vi "外观 2.vi"(0 "Data In":T4 caption="数据输入", 2 "Display State In":T2 caption="显示状态输入", 3 "Container State":T3 caption="容器状态") -> (6 "Data Out":T4 caption="数据输出", 7 "Display State Out":T2 caption="显示状态输出", 8 "Action":T1 caption="动作")   [LabVIEW 2016, in "多参数测量数据.xctl"]
uses:
  <vilib>/_xctls/Container State.ctl
  <vilib>/_xctls/Action.ctl
  <vilib>/_xctls/XControlSupport.lvlib
panel:
  out "数据标识":string
  out "实测值":string
  out "数据时间":string
  out "单位":string
  out "因子编码":string
  # "因子编码:"
  # "单位:"
  # "数据时间:"
  # "实测值:"
  # "数据标识:"
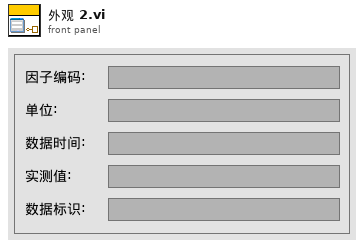
[diagram p1: front panel]
types:
  T1 = typedef "XControlSupport.lvlib/Action.ctl" = cluster{"Data Changed?":bool, "State Changed?":bool, "Action Name":string}
  T2 = typedef "多参数测量数据.xctl/状态 1.ctl" = cluster{"Numeric":dbl}
  T3 = typedef "XControlSupport.lvlib/Container State.ctl" = cluster{"Indicator?":bool, "Run Mode?":bool, " Refnum":refnum<vi>}
  T4 = typedef "多参数测量数据.xctl/数据 1.ctl" = cluster{"测量精度":u16, "测量数据区":cluster{"因子编码":string, "单位":string, "标样参考值":sgl, "水样数据时间":timestamp, "水样实测值":sgl, "水样数据标识":string, "K":sgl, "B":sgl, "T":sgl, "H":sgl, "水深":sgl}}
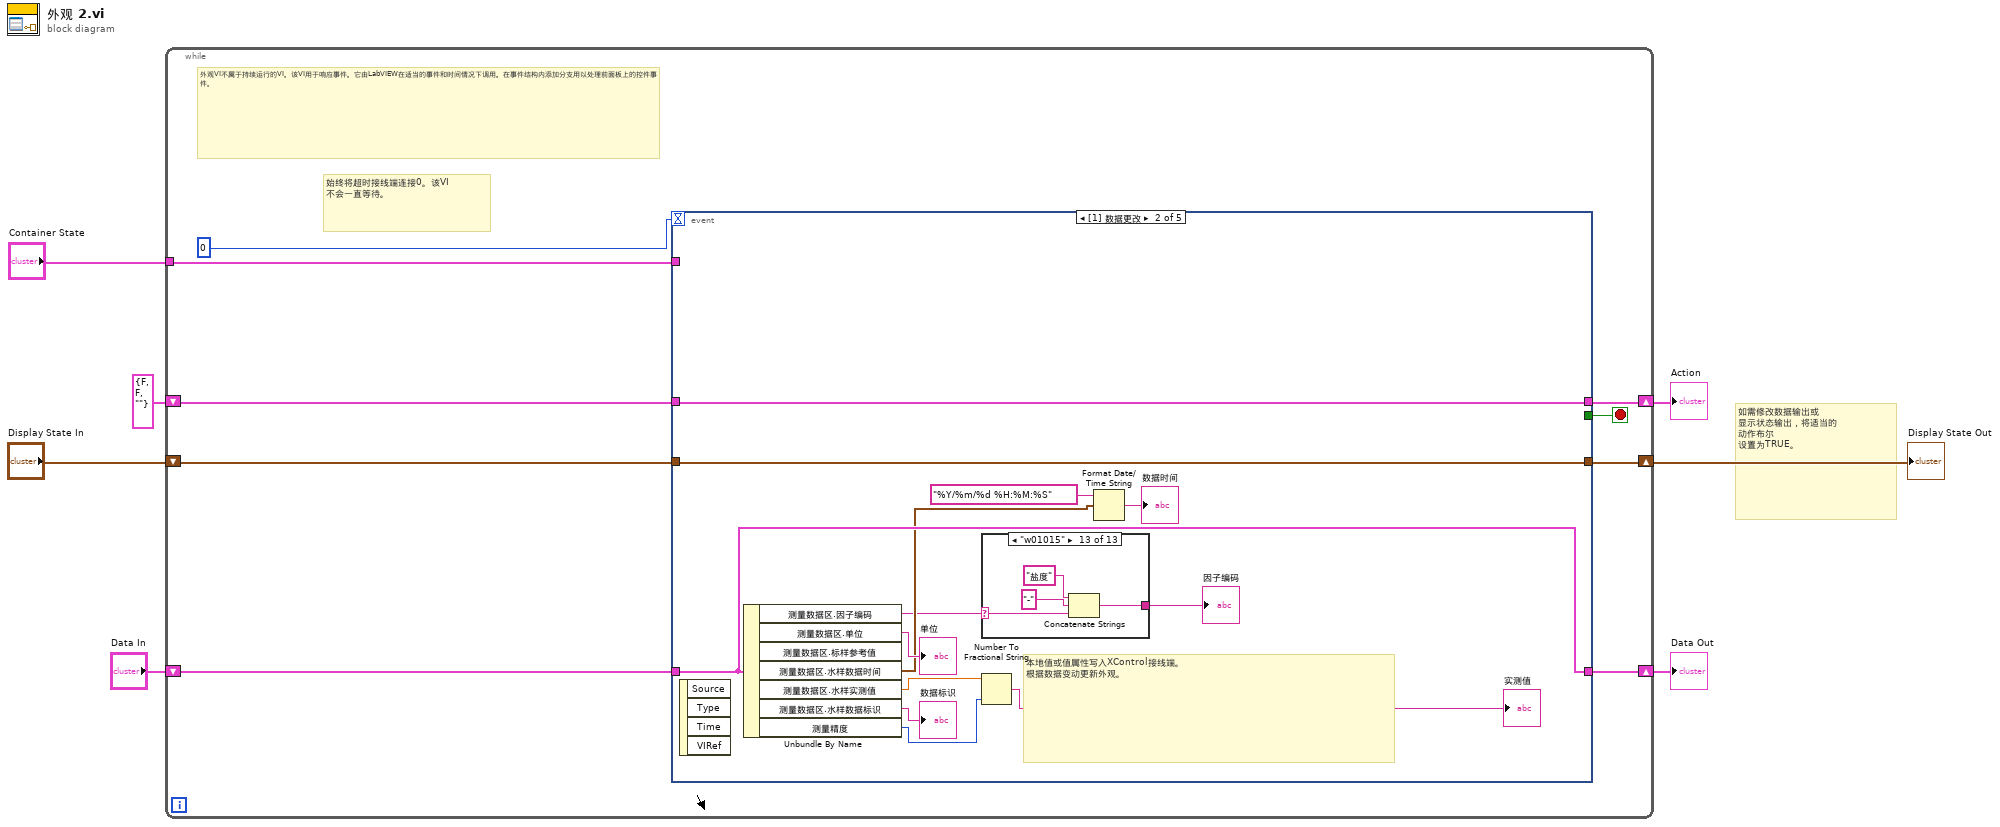
[diagram p0: block diagram]
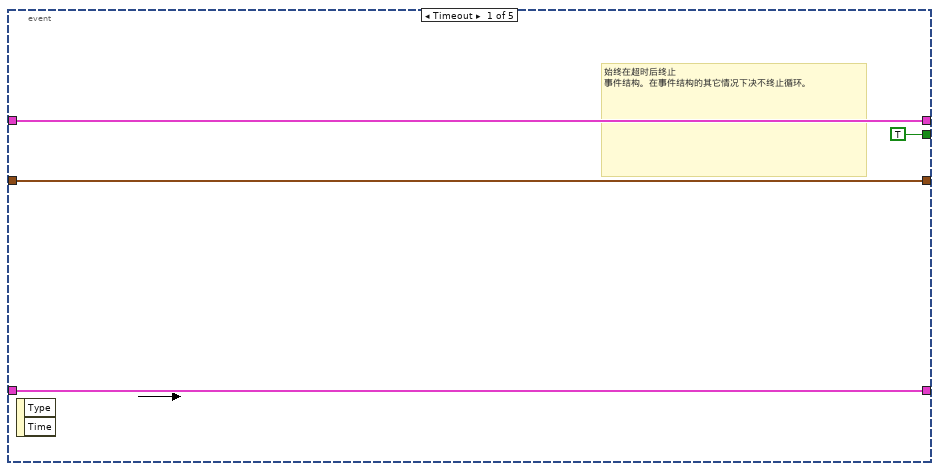
[diagram p2: hidden frame]
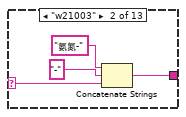
[diagram p4: hidden frame]
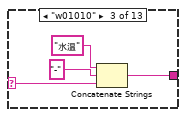
[diagram p5: hidden frame]
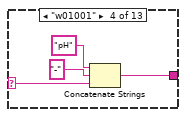
[diagram p6: hidden frame]
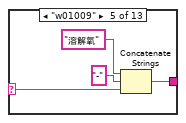
[diagram p7: hidden frame]
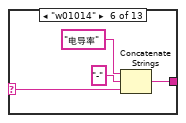
[diagram p8: hidden frame]
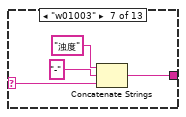
[diagram p9: hidden frame]
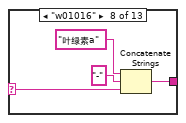
[diagram p10: hidden frame]
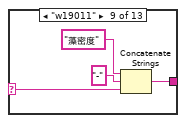
[diagram p11: hidden frame]
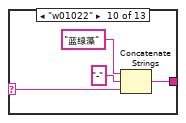
[diagram p12: hidden frame]
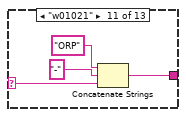
[diagram p13: hidden frame]
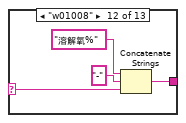
[diagram p14: hidden frame]
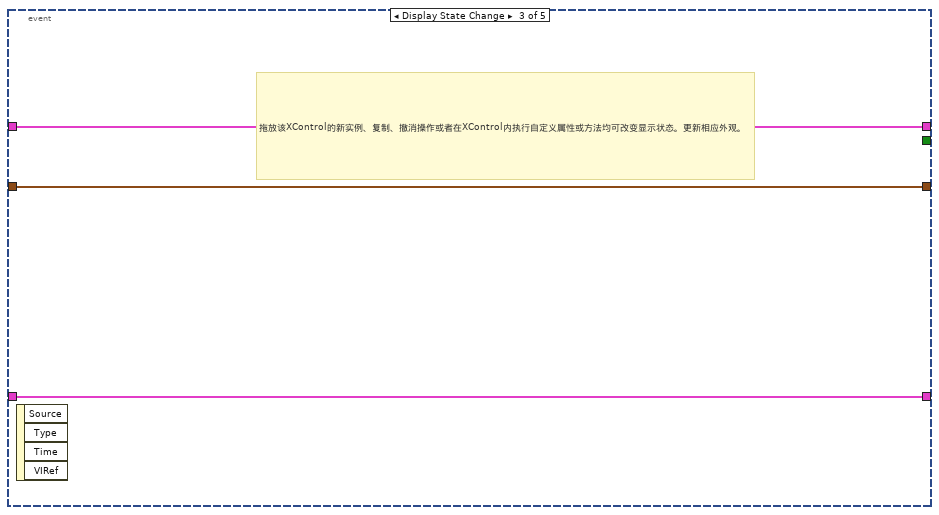
[diagram p15: hidden frame]
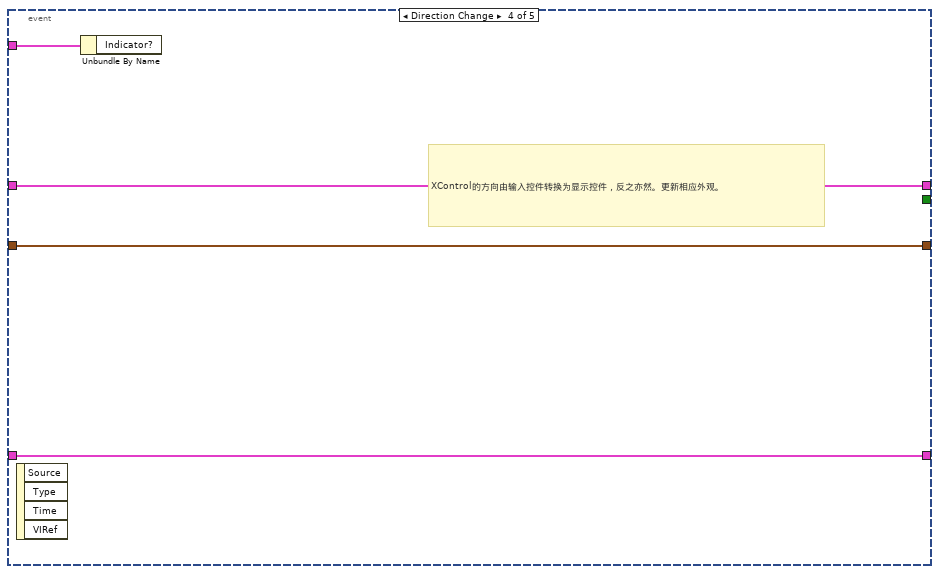
[diagram p16: hidden frame]
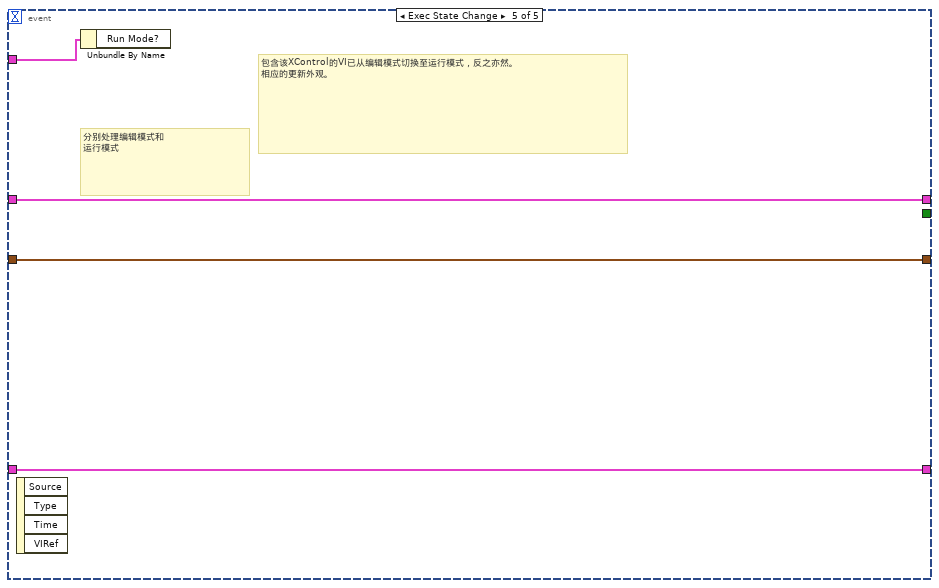
[diagram p17: hidden frame]
diagram:
  # "如需修改数据输出或\n显示状态输出，将适当的\n动作布尔\n设置为TRUE。"
  n1 = while {
    shift-right: [w15] -> w4
    shift-left: "Display State In" -> [w16]
    tunnel: "Container State" -> [w12]
    shift-right: [w10] -> w7
    shift-left: "Data In" -> [w11]
    shift-right: [w8] -> w2
    shift-left: T1 {"Data Changed?"=FALSE, "State Changed?"=FALSE, "Action Name"=""} ("Action") -> [w9]
    stop <- w14 stop-if-true
    # "外观VI不属于持续运行的VI。该VI用于响应事件。它由LabVIEW在适当的事件和时间情况下调用。在事件结构内添加分支用以处理前面板上的控件事件。"
    # "始终将超时接线端连接0。该VI\n不会一直等待。"
    n2 = event shown="[1] 数据更改" {
      selector: _ -> [_ _ _ _ _]
      dyn-events: _ -> [_ _ _ _ _]
      timeout: 0 -> [_ _ _ _ _]
      tunnel: w16 -> [w18 w33 w85 w88 w92]
      tunnel: [w18 w33 w85 w88 w92] -> w15
      tunnel: [TRUE _ _ _ _] -> w14
      tunnel: w12 -> [_ _ _ w89 w93]
      tunnel: w11 -> [w17 w31 w84 w87 w91]
      tunnel: [w17 w31 w84 w87 w91] -> w10
      tunnel: [w19 w32 w83 w86 w90] -> w8
      tunnel: w9 -> [w19 w32 w83 w86 w90]
      event Timeout {
        # "始终在超时后终止\n事件结构。在事件结构的其它情况下决不终止循环。"
        n3 = event-data() -> ()  [unwired: 1 in, 2 out]
      }
      event Data Change {
        # "本地值或值属性写入XControl接线端。\n根据数据变动更新外观。"
        n4 = event-data() -> ()  [unwired: 1 in, 4 out]
        n5 = Unbundle By Name(w31) -> ("测量数据区.因子编码"=w23:string, "测量数据区.单位"=→"单位":string, "测量数据区.水样数据时间"=w25:timestamp, "测量数据区.水样实测值"=w27:sgl, "测量数据区.水样数据标识"=→"数据标识":string, "测量精度"=w21:u16)  [unwired: 1 out]
        n6 = case shown="\"w01015\"" w23 {
          selector: w23 -> [w34 w38 w42 w46 w50 w54 w58 w62 w66 w70 w74 w78 w82]
          tunnel: [w34 w36 w40 w44 w48 w52 w56 w60 w64 w68 w72 w76 w80] -> w22
          frame Default {
          }
          frame "w21003" {
            n7 = Concatenate Strings("氨氮-" ("字符串"), "-" ("字符串"), w38) -> (w36:string)
          }
          frame "w01010" {
            n8 = Concatenate Strings("水温" ("字符串"), "-" ("字符串"), w42) -> (w40:string)
          }
          frame "w01001" {
            n9 = Concatenate Strings("pH" ("字符串"), "-" ("字符串"), w46) -> (w44:string)
          }
          frame "w01009" {
            n10 = Concatenate Strings("溶解氧" ("字符串"), "-" ("字符串"), w50) -> (w48:string)
          }
          frame "w01014" {
            n11 = Concatenate Strings("电导率" ("字符串"), "-" ("字符串"), w54) -> (w52:string)
          }
          frame "w01003" {
            n12 = Concatenate Strings("浊度" ("字符串"), "-" ("字符串"), w58) -> (w56:string)
          }
          frame "w01016" {
            n13 = Concatenate Strings("叶绿素a" ("字符串"), "-" ("字符串"), w62) -> (w60:string)
          }
          frame "w19011" {
            n14 = Concatenate Strings("藻密度" ("字符串"), "-" ("字符串"), w66) -> (w64:string)
          }
          frame "w01022" {
            n15 = Concatenate Strings("蓝绿藻" ("字符串"), "-" ("字符串"), w70) -> (w68:string)
          }
          frame "w01021" {
            n16 = Concatenate Strings("ORP" ("字符串"), "-" ("字符串"), w74) -> (w72:string)
          }
          frame "w01008" {
            n17 = Concatenate Strings("溶解氧%" ("字符串"), "-" ("字符串"), w78) -> (w76:string)
          }
          frame "w01015" {
            n18 = Concatenate Strings("盐度" ("字符串"), "-" ("字符串"), w82) -> (w80:string)
          }
        }
        "因子编码" <- w22
        n19 = Number To Fractional String(number=w27, precision (6)=w21) -> (F-format string=→"实测值":string)  [unwired: 2 in]
        n20 = Format Date/Time String(time format string (%c)="%Y/%m/%d %H:%M:%S" ("时间格式字符串(%c)"), seconds (now)=w25) -> (date/time string=→"数据时间":string)  [unwired: 1 in]
      }
      event Display State Change {
        # "拖放该XControl的新实例、复制、撤消操作或者在XControl内执行自定义属性或方法均可改变显示状态。更新相应外观。"
        n21 = event-data() -> ()  [unwired: 1 in, 4 out]
      }
      event Direction Change {
        # "XControl的方向由输入控件转换为显示控件，反之亦然。更新相应外观。"
        n22 = event-data() -> ()  [unwired: 1 in, 4 out]
        n23 = Unbundle By Name(w89) -> ()  [unwired: 1 out]
      }
      event Exec State Change {
        # "包含该XControl的VI已从编辑模式切换至运行模式，反之亦然。\n相应的更新外观。"
        # "分别处理编辑模式和\n运行模式"
        n24 = event-data() -> ()  [unwired: 1 in, 4 out]
        n25 = Unbundle By Name(w93) -> ()  [unwired: 1 out]
      }
    }
  }
  "Display State Out" <- w4
  "Data Out" <- w7
  "Action" <- w2
